vi "Create AppEvent Queue.vi"(8 "Error In":errorcluster, 11 "EventLog in":refnum<class "EventLog.lvclass">) -> (0 "Error Out":errorcluster, 3 "EventLog out":refnum<class "EventLog.lvclass">)   [LabVIEW 2019, in "EventLog.lvlib" / "EventLog.lvclass"]
uses:
  EventLog.lvclass
  Classes/Events/Events.lvclass
  EventLog.lvclass/EventLog.ctl
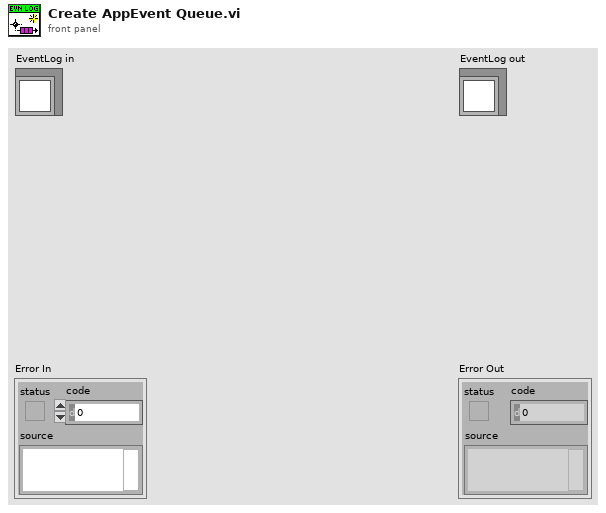
[diagram p1: front panel]
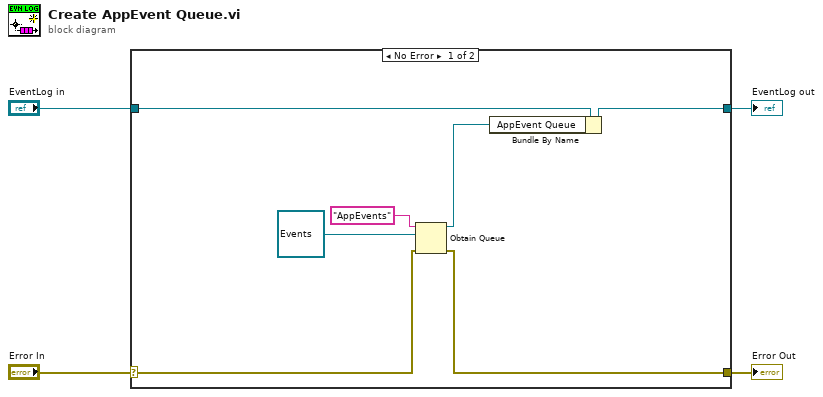
[diagram p0: block diagram]
diagram:
  n1 = case shown="No Error" "Error In" {
    selector: "Error In" -> [w8 w13]
    tunnel: [w7 w13] -> w3
    tunnel: [w6 w12] -> w1
    tunnel: "EventLog in" -> [w11 w12]
    frame No Error {
      n2 = Obtain Queue(name (unnamed)="AppEvents", element data type=refnum<class "Events.lvclass"> refnum ("Events.lvclass"), error in (no error)=w8) -> (queue out=w5:refnum<queue>, error out=w7:errorcluster)  [unwired: 2 in, 1 out]
      n3 = Bundle By Name(cluster=w11, "AppEvent Queue"=w5) -> (w6:refnum<class "EventLog.lvclass">)
    }
    frame Error {
    }
  }
  "Error Out" <- w3
  "EventLog out" <- w1
